vi "goto.vi"(2 "Numeric 3":sgl=-100.0, 3 "Numeric":sgl=-100.0, 4 "Numeric 2":sgl=-100.0, 5 "error out 2":errorcluster, 6 "new element/subarray":i32=1, 7 "VISA resource name 2":refnum<visa-resource-name>) -> (0 "error out 3":errorcluster, 1 "VISA resource name 3":refnum<visa-resource-name>)   [LabVIEW 2017]
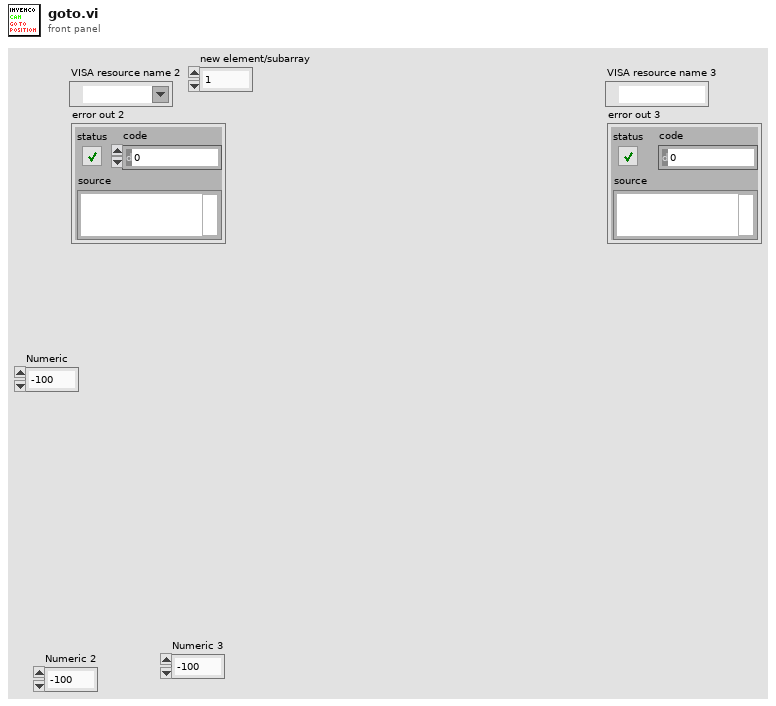
[diagram p1: front panel]
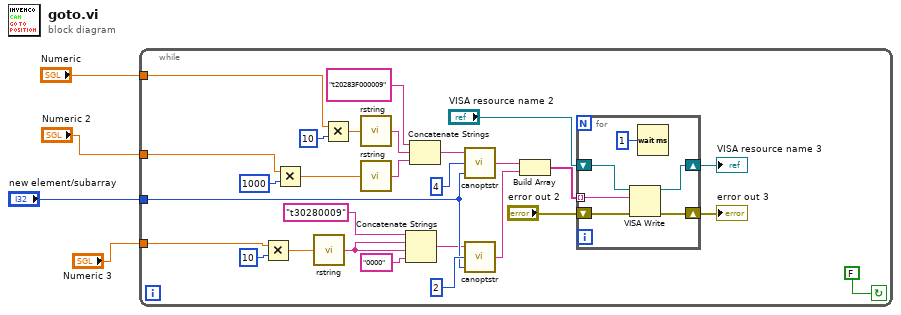
[diagram p0: block diagram]
diagram:
  n1 = while {
    tunnel: "new element/subarray" -> [w22]
    tunnel: "Numeric 2" -> [w7]
    tunnel: "Numeric 3" -> [w6]
    tunnel: "Numeric" -> [w5]
    stop <- FALSE continue-if-true
    n2 = Multiply(x=w6, y=i16 10) -> (x*y=w14:sgl)
    n3 = Multiply(x=w7, y=i16 1000) -> (x*y=w16:sgl)
    n4 = call "rstring.vi"("number"=w14) -> ("concatenated string"=w11:string)
    n5 = Multiply(x=w5, y=i16 10) -> (x*y=w19:sgl)
    n6 = call "rstring.vi"("number"=w19) -> ("concatenated string"=w18:string)
    n7 = call "rstring.vi"("number"=w16) -> ("concatenated string"=w15:string)
    n8 = Concatenate Strings("t30280009", w11, w11, "0000" ("string")) -> (w8:string)
    n9 = Concatenate Strings("t20283F000009", w18, w15) -> (w9:string)
    n10 = call "canoptstr.vi"("new element/subarray"=w22, "index"=4, "String 2"=w9) -> ("String"=w26:string)
    n11 = call "canoptstr.vi"("new element/subarray"=w22, "index"=2, "String 2"=w8) -> ("String"=w27:string)
    n12 = Build Array(w26, w27) -> (w23:string[])
    n13 = for {
      tunnel: w23 -> [w34] mode=indexing
      shift-right: [w36] -> w32
      shift-left: "VISA resource name 2" -> [w38]
      shift-right: [w35] -> w31
      shift-left: "error out 2" -> [w37]
      n14 = VISA Write(VISA resource name=w38, write buffer=w34, error in (no error)=w37) -> (VISA resource name out=w36:refnum<visa-resource-name>, error out=w35:errorcluster)  [unwired: 1 out]
      n15 = Wait (ms)(milliseconds to wait=u32 1 ("millisecond multiple")) -> ()  [unwired: 1 out]
    }
    "VISA resource name 3" <- w32
    "error out 3" <- w31
  }
